vi "Read FIFO Payload Length.vi"(8 "error in (no error)":errorcluster, 11 "CIFChannels in":refnum<class "CIFChannels.lvclass">) -> (0 "error out":errorcluster, 2 "Payload Length":u64, 3 "CIFChannels out":refnum<class "CIFChannels.lvclass">)   [LabVIEW 2021, in "CIFChannels.lvclass"]
uses:
  CIFChannels.lvclass
  CIFChannels.lvclass/CIFChannels.ctl
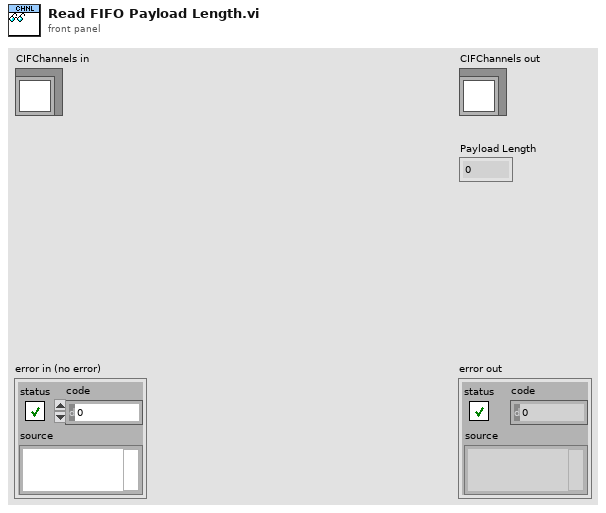
[diagram p1: front panel]
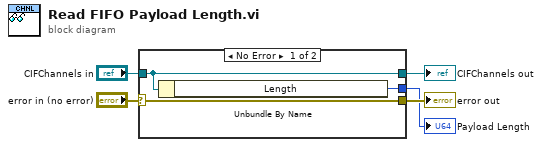
[diagram p0: block diagram]
diagram:
  n1 = case shown="No Error" "error in (no error)" {
    selector: "error in (no error)" -> [w8 w9]
    tunnel: [w8 w9] -> w4
    tunnel: [w7 w10] -> w2
    tunnel: "CIFChannels in" -> [w7 w10]
    tunnel: [w6 _] -> w1
    frame No Error {
      n2 = Unbundle By Name(w7) -> ("Length"=w6:u64)
    }
    frame Error {
    }
  }
  "error out" <- w4
  "CIFChannels out" <- w2
  "Payload Length" <- w1
